vi "writeToXML.vi"(8 "error in (no error)":errorcluster, 10 "ClassLabel":string, 11 "MccReference in":refnum<class "MccReference.lvclass">) -> (0 "error out":errorcluster, 2 "XML out":string, 3 "MccReference out":refnum<class "MccReference.lvclass">)   [LabVIEW 2022 SP3, in "TCSDataDefinitions.lvlib" / "TCSMountControlCommand.lvlib" / "CommandsForAllAxes.lvlib" / "MccReference.lvclass"]
uses:
  MccReference.lvclass
  CommandsForAllAxes.lvclass
  <userlib>/Common/XML/XMLGenerator/XMLGenerator.lvclass
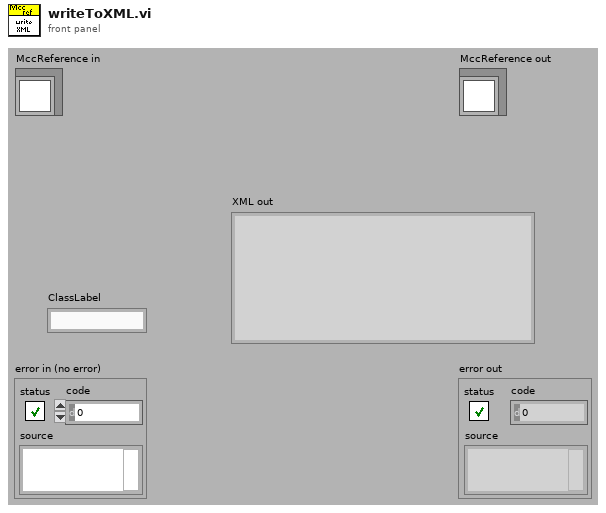
[diagram p1: front panel]
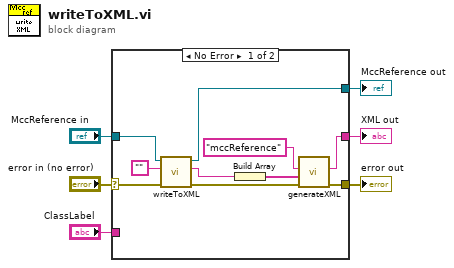
[diagram p0: block diagram]
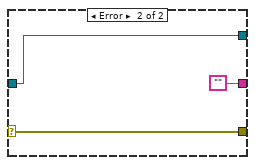
[diagram p2: hidden frame]
diagram:
  n1 = case shown="No Error" "error in (no error)" {
    selector: "error in (no error)" -> [w9 w19]
    tunnel: [w8 w19] -> w5
    tunnel: [w15 w18] -> w3
    tunnel: "MccReference in" -> [w16 w18]
    tunnel: [w10 ""] -> w2
    tunnel: "ClassLabel" -> [_ _]
    frame No Error {
      n2 = call-parent "writeToXML.vi"("error in (no error)"=w9, "ClassLabel"="", "CommandsForAllAxes in"=w16) -> ("error out"=w7:errorcluster, "XMLout"=w13:string, "CommandsForAllAxes out"=w15:refnum<class "MccReference.lvclass">)  [unwired: 6 in]
      n3 = Build Array(w13) -> (w12:string[])
      n4 = call <userlib>:"generateXML.vi"("error in"=w7, "childrenXML"=w12, "elementName"="mccReference" ("Class Label")) -> ("error out"=w8:errorcluster, "XML out"=w10:string)  [unwired: 6 in, 1 out]
    }
    frame Error {
    }
  }
  "error out" <- w5
  "MccReference out" <- w3
  "XML out" <- w2
